vi "BCtr5.vi"() -> ()   [LabVIEW 2016]
uses:
  <vilib>/platform/TimedLoop/XDataNode/XDataNode.xnode
  <vilib>/Platform/TimedLoop/XDataNode/nitl_modes.ctl
  <vilib>/Platform/TimedLoop/XDataNode/XDNodeRunTimeDep.lvlib
  <vilib>/Platform/TimedLoop/XDataNode/wakeup.ctl
  <vilib>/Platform/TimedLoop/XDataNode/timing_clust.ctl
panel:
  in  "CtrEn":bool
  out "Waveform Chart":u16(graph)
  out "LoopCt":dbl
  out "Ack":bool
  out "error out":errorcluster
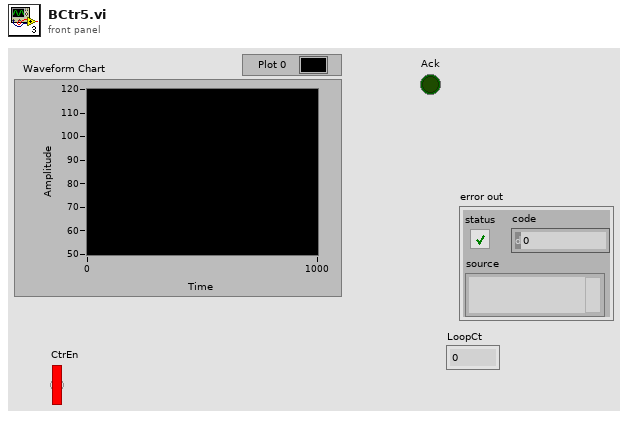
[diagram p1: front panel]
types:
  T1 = cluster{"Nbins":u16, "BaseAddrOut":u16, "PortOut":string, "ConfigOK":bool, "MreadFmt":string}
  T2 = typedef "XDNodeRunTimeDep.lvlib/timing_clust.ctl" = cluster{"Expected End [f-1]":u64, "Actual End [f-1]":u64, "Finished Late? [f-1]":bool, "Expected End [i-1]":u64, "Actual End [i-1]":u64, "Finished Late? [i-1]":bool, "Expected Start [i]":u64, "Actual Start [i]":u64, "Expected Start [f]":u64, "Actual Start [f]":u64, "Source Name":string, "Structure Name":string, "Period":i64, "Deadline":i64, "Offset":i64, "Start":i64, "Priority":i32, "Timeout":i32, "Mode":T3, "Wakeup Reason":T4, "Error":errorcluster, "Source Type":string, "Secondary Source Type":string, "Global End Time":u64, "Global Start Time":u64, "Frame Duration":u64, "Iteration Duration":u64, "Assigned CPU":i32, "I/O Scan Engine Mode":u32}
  T3 = typedef "XDNodeRunTimeDep.lvlib/nitl_modes.ctl" = enum32{"No Change", "Process missed periods, maintain original phase", "Discard missed periods, maintain original phase", "Process missed periods, ignore original phase", "Discard missed periods, ignore original phase"}
  T4 = typedef "XDNodeRunTimeDep.lvlib/wakeup.ctl" = enum32{"Normal", "Aborted", "Asynchronous wakeup", "Timing source error", "Timed loop error", "Timeout"}
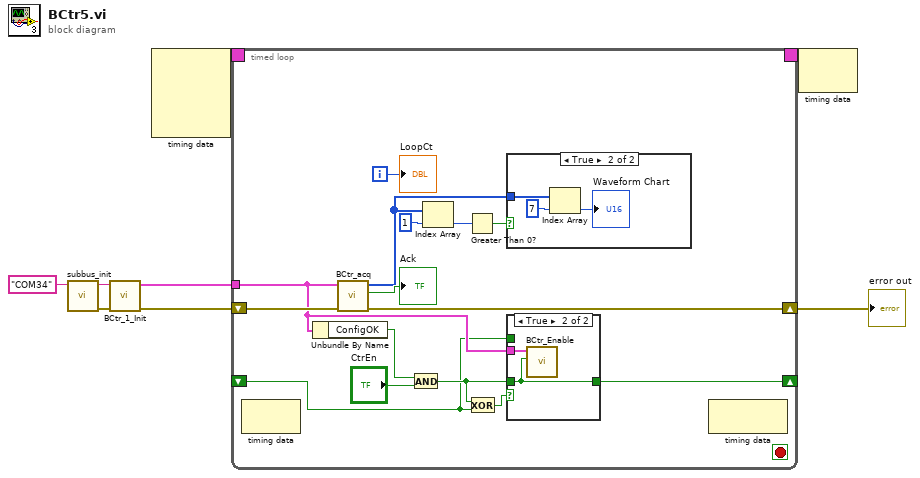
[diagram p0: block diagram]
diagram:
  n1 = call "subbus_init.vi"("Port"="COM34") -> ("error out"=w3:errorcluster, "PortOut"=w4:string)  [unwired: 9 in]
  n2 = call "BCtr_1_Init.vi"("error in (no error)"=w3, "SBPort"=w4) -> ("error out"=w2:errorcluster, "CtrCfg"=w1:T1)  [unwired: 8 in]
  n3 = node-c288() -> (w6:T2)  [unwired: 4 in]
  n4 = timed-loop {
    timing: w6 -> [_]
    timing-out: [_] -> w5
    shift-right: [w22] -> w7
    shift-left: w2 -> [w23]
    tunnel: w1 -> [w12]
    shift-right: [w10] -> _
    shift-left: _ -> [w9]
    i -> [w20]
    stop <- _ stop-if-true
    n5 = node-c288() -> ()  [unwired: 1 in, 1 out]
    n6 = Unbundle By Name(w12) -> ("ConfigOK"=w15:bool)
    n7 = call "BCtr_acq.vi"("error in (no error)"=w23, "CtrCfg"=w12) -> ("error out"=w22:errorcluster, "Ack"=→"Ack":bool, "Values"=w19:u16[])  [unwired: 7 in]
    n8 = And(x=w15, y="CtrEn") -> (x .and. y?=w11:bool)
    n9 = Index Array(array=w19, index=1) -> (element=w17:u16)
    n10 = Greater Than 0?(x=w17) -> (x > 0?=w16:bool)
    n11 = Exclusive Or(1:w9, 2:w11) -> (0:w13:bool)
    n12 = case shown="True" w16 {
      tunnel: w19 -> [_ w29]
      frame False {
      }
      frame True {
        n13 = Index Array(array=w29, index=7) -> (element=→"Waveform Chart":u16)
      }
    }
    n14 = case shown="True" w13 {
      tunnel: w12 -> [_ w26]
      tunnel: w11 -> [_ w25]
      tunnel: [w24 w25] -> w10
      tunnel: w9 -> [w24 _]
      frame False {
      }
      frame True {
        n15 = call "BCtr_Enable.vi"("Enable"=w25, "CtrCfg"=w26) -> ()  [unwired: 8 in, 2 out]
      }
    }
    n16 = node-c288() -> ()  [unwired: 1 in, 1 out]
    "LoopCt" <- w20
  }
  "error out" <- w7
  n17 = node-c288(w5) -> ()  [unwired: 1 out]
